vi "Motor_generatespeed.vi"(2 "error in (no error)":errorcluster, 3 "Conversion\n (steps/mm)":dbl[](array[numeric])=[12500.0, 31496.063, 31496.063] format="%#_13g", 4 "Speed (mm/s)":dbl[](array[numeric]) format="%#_13g", 5 "reference":refnum<k7>) -> (0 "error out":errorcluster, 1 "reference out":refnum<k7>)   [LabVIEW 2018]
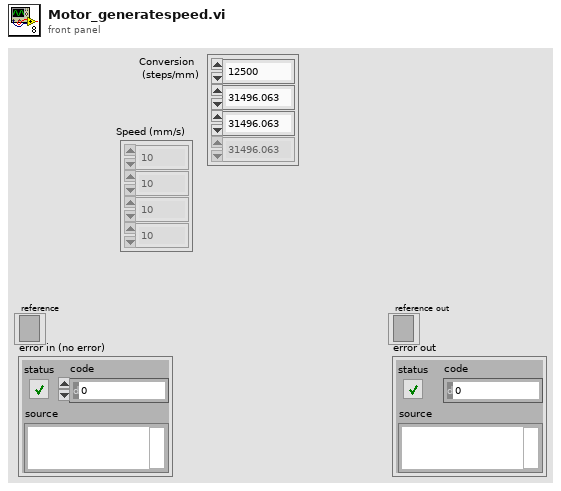
[diagram p1: front panel]
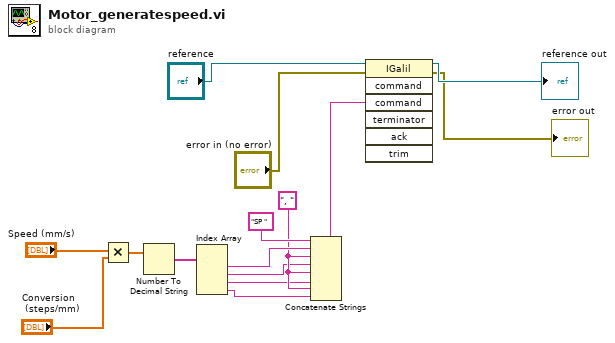
[diagram p0: block diagram]
diagram:
  w4 = ", " ("string")
  n1 = Multiply(x="Speed (mm/s)", y="Conversion\n (steps/mm)") -> (x*y=w11:dbl[])
  n2 = Number To Decimal String(number=w11) -> (decimal integer string=w5:string[])  [unwired: 1 in]
  n3 = Index Array(array=w5) -> (element #1=w15:string, element #2=w3:string, element #3=w2:string, element #4=w1:string)  [unwired: 4 in]
  n4 = Concatenate Strings("SP " ("string"), w15, w4, w3, w4, w2, w4, w1) -> (w6:string)
  n5 = invoke class="IGalil" method="command"(reference="reference", error in="error in (no error)", "command"=w6) -> (reference out=→"reference out":refnum<k7>, error out=→"error out":errorcluster)  [unwired: 4 in, 5 out]
